vi "simplegit.TortoiseGitProc.vi"() -> (3 "Path":path)   [LabVIEW 2017]
uses:
  <resource>/dialog/lvconfig.llb/LV Config Read Pathlist.vi
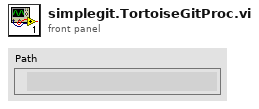
[diagram p1: front panel]
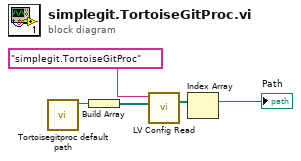
[diagram p0: block diagram]
diagram:
  n1 = call "Tortoisegitproc default path.vi"() -> ("TortoiseGitProc.exe"=w5:path)  [unwired: 10 in, 1 out]
  n2 = Build Array(w5) -> (w1:path[])
  n3 = call-poly <resource>:"LV Config Read.vi"("default value"=w1, "key"="simplegit.TortoiseGitProc") -> ("value"=w3:path[])  [unwired: 3 in, 2 out]
  n4 = Index Array(array=w3) -> (element=→"Path":path)  [unwired: 1 in]
